vi "ActiView806-Lores.vi"() -> ()   [LabVIEW 2020] (continued)
                      tunnel: w4514 -> [w4583 w4585 w4587 w4589 w4591 w4593 w4595 w4597 w4599 w4601 w4603 w4605 w4607 w4609 w4611 w4613 w4615 w4617 w4619 w4621 w4623 w4625 w4627 w4629 w4631 w4633 w4635 w4637 w4639 w4641 w4643 w4645 w4647 w4649 w4651 w4653 w4655 w4657 w4659 w4661 w4663 w4665 w4667 w4669 w4671 w4673 w4675 w4677 w4679 w4681 w4683 w4685 w4687 w4689 w4691 w4693 w4695 w4697 w4699 w4701 w4703 w4705 w4707 w4709]
                      frame 1 {
                        n1833 = property on="Trace1" class="Str"("Position:Top"=w4583) -> ()  [unwired: 2 in, 2 out]
                        "Trace1" <- w4584
                      }
                      frame 2 {
                        n1834 = property on="Trace2" class="Str"("Position:Top"=w4585) -> ()  [unwired: 2 in, 2 out]
                        "Trace2" <- w4586
                      }
                      frame 3 {
                        n1835 = property on="Trace3" class="Str"("Position:Top"=w4587) -> ()  [unwired: 2 in, 2 out]
                        "Trace3" <- w4588
                      }
                      frame 4 {
                        n1836 = property on="Trace4" class="Str"("Position:Top"=w4589) -> ()  [unwired: 2 in, 2 out]
                        "Trace4" <- w4590
                      }
                      frame 5 {
                        n1837 = property on="Trace5" class="Str"("Position:Top"=w4591) -> ()  [unwired: 2 in, 2 out]
                        "Trace5" <- w4592
                      }
                      frame 6 {
                        n1838 = property on="Trace6" class="Str"("Position:Top"=w4593) -> ()  [unwired: 2 in, 2 out]
                        "Trace6" <- w4594
                      }
                      frame 7 {
                        n1839 = property on="Trace7" class="Str"("Position:Top"=w4595) -> ()  [unwired: 2 in, 2 out]
                        "Trace7" <- w4596
                      }
                      frame 8 {
                        n1840 = property on="Trace8" class="Str"("Position:Top"=w4597) -> ()  [unwired: 2 in, 2 out]
                        "Trace8" <- w4598
                      }
                      frame 9 {
                        n1841 = property on="Trace9" class="Str"("Position:Top"=w4599) -> ()  [unwired: 2 in, 2 out]
                        "Trace9" <- w4600
                      }
                      frame 10 {
                        n1842 = property on="Trace10" class="Str"("Position:Top"=w4601) -> ()  [unwired: 2 in, 2 out]
                        "Trace10" <- w4602
                      }
                      frame 11 {
                        n1843 = property on="Trace11" class="Str"("Position:Top"=w4603) -> ()  [unwired: 2 in, 2 out]
                        "Trace11" <- w4604
                      }
                      frame 12 {
                        n1844 = property on="Trace12" class="Str"("Position:Top"=w4605) -> ()  [unwired: 2 in, 2 out]
                        "Trace12" <- w4606
                      }
                      frame 13 {
                        n1845 = property on="Trace13" class="Str"("Position:Top"=w4607) -> ()  [unwired: 2 in, 2 out]
                        "Trace13" <- w4608
                      }
                      frame 14 {
                        n1846 = property on="Trace14" class="Str"("Position:Top"=w4609) -> ()  [unwired: 2 in, 2 out]
                        "Trace14" <- w4610
                      }
                      frame 15 {
                        n1847 = property on="Trace15" class="Str"("Position:Top"=w4611) -> ()  [unwired: 2 in, 2 out]
                        "Trace15" <- w4612
                      }
                      frame 16 {
                        n1848 = property on="Trace16" class="Str"("Position:Top"=w4613) -> ()  [unwired: 2 in, 2 out]
                        "Trace16" <- w4614
                      }
                      frame 17 {
                        n1849 = property on="Trace17" class="Str"("Position:Top"=w4615) -> ()  [unwired: 2 in, 2 out]
                        "Trace17" <- w4616
                      }
                      frame 18 {
                        n1850 = property on="Trace18" class="Str"("Position:Top"=w4617) -> ()  [unwired: 2 in, 2 out]
                        "Trace18" <- w4618
                      }
                      frame 19 {
                        n1851 = property on="Trace19" class="Str"("Position:Top"=w4619) -> ()  [unwired: 2 in, 2 out]
                        "Trace19" <- w4620
                      }
                      frame 20 {
                        n1852 = property on="Trace20" class="Str"("Position:Top"=w4621) -> ()  [unwired: 2 in, 2 out]
                        "Trace20" <- w4622
                      }
                      frame 21 {
                        n1853 = property on="Trace21" class="Str"("Position:Top"=w4623) -> ()  [unwired: 2 in, 2 out]
                        "Trace21" <- w4624
                      }
                      frame 22 {
                        n1854 = property on="Trace22" class="Str"("Position:Top"=w4625) -> ()  [unwired: 2 in, 2 out]
                        "Trace22" <- w4626
                      }
                      frame 23 {
                        n1855 = property on="Trace23" class="Str"("Position:Top"=w4627) -> ()  [unwired: 2 in, 2 out]
                        "Trace23" <- w4628
                      }
                      frame 24 {
                        n1856 = property on="Trace24" class="Str"("Position:Top"=w4629) -> ()  [unwired: 2 in, 2 out]
                        "Trace24" <- w4630
                      }
                      frame 25 {
                        n1857 = property on="Trace25" class="Str"("Position:Top"=w4631) -> ()  [unwired: 2 in, 2 out]
                        "Trace25" <- w4632
                      }
                      frame 26 {
                        n1858 = property on="Trace26" class="Str"("Position:Top"=w4633) -> ()  [unwired: 2 in, 2 out]
                        "Trace26" <- w4634
                      }
                      frame 27 {
                        n1859 = property on="Trace27" class="Str"("Position:Top"=w4635) -> ()  [unwired: 2 in, 2 out]
                        "Trace27" <- w4636
                      }
                      frame 28 {
                        n1860 = property on="Trace28" class="Str"("Position:Top"=w4637) -> ()  [unwired: 2 in, 2 out]
                        "Trace28" <- w4638
                      }
                      frame 29 {
                        n1861 = property on="Trace29" class="Str"("Position:Top"=w4639) -> ()  [unwired: 2 in, 2 out]
                        "Trace29" <- w4640
                      }
                      frame 30 {
                        n1862 = property on="Trace30" class="Str"("Position:Top"=w4641) -> ()  [unwired: 2 in, 2 out]
                        "Trace30" <- w4642
                      }
                      frame 31 {
                        n1863 = property on="Trace31" class="Str"("Position:Top"=w4643) -> ()  [unwired: 2 in, 2 out]
                        "Trace31" <- w4644
                      }
                      frame 32 {
                        n1864 = property on="Trace32" class="Str"("Position:Top"=w4645) -> ()  [unwired: 2 in, 2 out]
                        "Trace32" <- w4646
                      }
                      frame 33 {
                        n1865 = property on="Trace33" class="Str"("Position:Top"=w4647) -> ()  [unwired: 2 in, 2 out]
                        "Trace33" <- w4648
                      }
                      frame 34 {
                        n1866 = property on="Trace34" class="Str"("Position:Top"=w4649) -> ()  [unwired: 2 in, 2 out]
                        "Trace34" <- w4650
                      }
                      frame 35 {
                        n1867 = property on="Trace35" class="Str"("Position:Top"=w4651) -> ()  [unwired: 2 in, 2 out]
                        "Trace35" <- w4652
                      }
                      frame 36 {
                        n1868 = property on="Trace36" class="Str"("Position:Top"=w4653) -> ()  [unwired: 2 in, 2 out]
                        "Trace36" <- w4654
                      }
                      frame 37 {
                        n1869 = property on="Trace37" class="Str"("Position:Top"=w4655) -> ()  [unwired: 2 in, 2 out]
                        "Trace37" <- w4656
                      }
                      frame 38 {
                        n1870 = property on="Trace38" class="Str"("Position:Top"=w4657) -> ()  [unwired: 2 in, 2 out]
                        "Trace38" <- w4658
                      }
                      frame 39 {
                        n1871 = property on="Trace39" class="Str"("Position:Top"=w4659) -> ()  [unwired: 2 in, 2 out]
                        "Trace39" <- w4660
                      }
                      frame 40 {
                        n1872 = property on="Trace40" class="Str"("Position:Top"=w4661) -> ()  [unwired: 2 in, 2 out]
                        "Trace40" <- w4662
                      }
                      frame 41 {
                        n1873 = property on="Trace41" class="Str"("Position:Top"=w4663) -> ()  [unwired: 2 in, 2 out]
                        "Trace41" <- w4664
                      }
                      frame 42 {
                        n1874 = property on="Trace42" class="Str"("Position:Top"=w4665) -> ()  [unwired: 2 in, 2 out]
                        "Trace42" <- w4666
                      }
                      frame 43 {
                        n1875 = property on="Trace43" class="Str"("Position:Top"=w4667) -> ()  [unwired: 2 in, 2 out]
                        "Trace43" <- w4668
                      }
                      frame 44 {
                        n1876 = property on="Trace44" class="Str"("Position:Top"=w4669) -> ()  [unwired: 2 in, 2 out]
                        "Trace44" <- w4670
                      }
                      frame 45 {
                        n1877 = property on="Trace45" class="Str"("Position:Top"=w4671) -> ()  [unwired: 2 in, 2 out]
                        "Trace45" <- w4672
                      }
                      frame 46 {
                        n1878 = property on="Trace46" class="Str"("Position:Top"=w4673) -> ()  [unwired: 2 in, 2 out]
                        "Trace46" <- w4674
                      }
                      frame 47 {
                        n1879 = property on="Trace47" class="Str"("Position:Top"=w4675) -> ()  [unwired: 2 in, 2 out]
                        "Trace47" <- w4676
                      }
                      frame 48 {
                        n1880 = property on="Trace48" class="Str"("Position:Top"=w4677) -> ()  [unwired: 2 in, 2 out]
                        "Trace48" <- w4678
                      }
                      frame 49 {
                        n1881 = property on="Trace49" class="Str"("Position:Top"=w4679) -> ()  [unwired: 2 in, 2 out]
                        "Trace49" <- w4680
                      }
                      frame 50 {
                        n1882 = property on="Trace50" class="Str"("Position:Top"=w4681) -> ()  [unwired: 2 in, 2 out]
                        "Trace50" <- w4682
                      }
                      frame 51 {
                        n1883 = property on="Trace51" class="Str"("Position:Top"=w4683) -> ()  [unwired: 2 in, 2 out]
                        "Trace51" <- w4684
                      }
                      frame 52 {
                        n1884 = property on="Trace52" class="Str"("Position:Top"=w4685) -> ()  [unwired: 2 in, 2 out]
                        "Trace52" <- w4686
                      }
                      frame 53 {
                        n1885 = property on="Trace53" class="Str"("Position:Top"=w4687) -> ()  [unwired: 2 in, 2 out]
                        "Trace53" <- w4688
                      }
                      frame 54 {
                        n1886 = property on="Trace54" class="Str"("Position:Top"=w4689) -> ()  [unwired: 2 in, 2 out]
                        "Trace54" <- w4690
                      }
                      frame 55 {
                        n1887 = property on="Trace55" class="Str"("Position:Top"=w4691) -> ()  [unwired: 2 in, 2 out]
                        "Trace55" <- w4692
                      }
                      frame 56 {
                        n1888 = property on="Trace56" class="Str"("Position:Top"=w4693) -> ()  [unwired: 2 in, 2 out]
                        "Trace56" <- w4694
                      }
                      frame 57 {
                        n1889 = property on="Trace57" class="Str"("Position:Top"=w4695) -> ()  [unwired: 2 in, 2 out]
                        "Trace57" <- w4696
                      }
                      frame 58 {
                        n1890 = property on="Trace58" class="Str"("Position:Top"=w4697) -> ()  [unwired: 2 in, 2 out]
                        "Trace58" <- w4698
                      }
                      frame 59 {
                        n1891 = property on="Trace59" class="Str"("Position:Top"=w4699) -> ()  [unwired: 2 in, 2 out]
                        "Trace59" <- w4700
                      }
                      frame 60 {
                        n1892 = property on="Trace60" class="Str"("Position:Top"=w4701) -> ()  [unwired: 2 in, 2 out]
                        "Trace60" <- w4702
                      }
                      frame 61 {
                        n1893 = property on="Trace61" class="Str"("Position:Top"=w4703) -> ()  [unwired: 2 in, 2 out]
                        "Trace61" <- w4704
                      }
                      frame 62 {
                        n1894 = property on="Trace62" class="Str"("Position:Top"=w4705) -> ()  [unwired: 2 in, 2 out]
                        "Trace62" <- w4706
                      }
                      frame 63 {
                        n1895 = property on="Trace63" class="Str"("Position:Top"=w4707) -> ()  [unwired: 2 in, 2 out]
                        "Trace63" <- w4708
                      }
                      frame 64, Default {
                        n1896 = property on="Trace64" class="Str"("Position:Top"=w4709) -> ()  [unwired: 2 in, 2 out]
                        "Trace64" <- w4710
                      }
                    }
                  }
                }
              }
              n1897 = Unbundle By Name(w3609) -> ("LoBatChange"=w3703:bool, "JazzLoBatChange"=w3362:bool)
              n1898 = Array Size(array=w3660) -> (size(s)=w3725:i32)
              n1899 = Array Size(array=w3414) -> (size(s)=w3590:i32)
              n1900 = Array Size(array=w3716) -> (size(s)=w3724:i32)
              n1901 = Array Size(array=w3695) -> (size(s)=w3697:i32)
              n1902 = property on="RefFree" class="LstBox (strict)"("Disabled"=w3726) -> ()  [unwired: 2 in, 2 out]
              n1903 = Unbundle By Name(w3394) -> ("Sweeping"=→"Sweeping":bool, "RejAbs"=→"RejAbs":bool, "RejDif"=→"RejDif":bool)
              n1904 = Not Equal?(x=w3725, y=w3724) -> (x != y?=w3721:bool)
              n1905 = Not Equal?(x=w3590, y=w3697) -> (x != y?=w3690:bool)
              n1906 = Not Equal?(x=w3660, y=w3716) -> (x != y?=w3723:bool[])
              n1907 = Not Equal?(x=w3414, y=w3695) -> (x != y?=w3696:bool[])
              n1908 = Or Array Elements(Boolean array=w3723) -> (logical OR=w3722:bool)
              n1909 = Or Array Elements(Boolean array=w3696) -> (logical OR=w3691:bool)
              n1910 = Compound Arithmetic op=OR(w3691, w3690, w3431) -> (w3689:bool)
              n1911 = case shown="True" w3689 {
                tunnel: w3448 -> [_ w4341]
                tunnel: w3414 -> [_ w4352]
                tunnel: w3590 -> [_ w4344]
                tunnel: w3381 -> [_ w4349]
                frame False {
                }
                frame True {
                  w4343 = 8  # Nr of Bip Labels
                  w4351 = -305.0  # Upper Y-value
                  w4354 = 519.0  # Lower Y-value
                  n1912 = Not Equal To 0?(x=w4344) -> (x != 0?=w4346:bool)
                  n1913 = Increment(x=w4344) -> (x+1=w4345:i32)
                  n1914 = Subtract(x=w4354, y=w4351) -> (x-y=w4353:dbl)
                  n1915 = Select(t=w4345, s=w4346, f=2) -> (s? t:f=w4342:i32)
                  n1916 = To Double Precision Float(number=w4342) -> (double precision float=w4348:dbl)
                  n1917 = Divide(x=w4353, y=w4348) -> (x/y=w4350:dbl)
                  n1918 = for {
                    N: w4343 -> [_]
                    tunnel: w4341 -> [w4359]
                    tunnel: w4352 -> [w4365]
                    tunnel: w4351 -> [w4362]
                    tunnel: w4350 -> [w4361]
                    tunnel: w4349 -> [w4363]
                    tunnel: w4344 -> [w4366]
                    i -> [w4364]
                    n1919 = Greater?(x=w4366, y=w4364) -> (0:w4356:bool)
                    n1920 = Increment(x=w4364) -> (x+1=w4360:i32)
                    n1921 = case shown="True" w4356 {
                      tunnel: w4362 -> [_ w4391]
                      tunnel: w4361 -> [_ w4390]
                      tunnel: w4359 -> [_ w4388]
                      tunnel: w4360 -> [_ w4383]
                      tunnel: ["" w4382] -> w4358
                      tunnel: [0 w4381] -> w4357
                      tunnel: w4363 -> [_ w4374]
                      tunnel: w4365 -> [_ w4380]
                      tunnel: w4364 -> [_ w4379]
                      frame False {
                      }
                      frame True {
                        w4384 = "\r"
                        w4387 = 4 ("length (rest)")
                        n1922 = Index Array(array=w4380, index=w4379) -> (element=w4371:i32)
                        n1923 = Increment(x=w4371) -> (x+1=w4370:i32)
                        n1924 = Less?(x=w4370, y=w4374) -> (x < y?=w4376:bool)
                        n1925 = Subtract(x=w4374, y=8) -> (x-y=w4372:i32)
                        n1926 = Select(t=w4370, s=w4376, f=w4372) -> (s? t:f=w4375:i32)
                        n1927 = To Double Precision Float(number=w4383) -> (double precision float=w4389:dbl)
                        n1928 = Index Array(array=w4388, index=w4371) -> (element=w4386:string)
                        n1929 = Index Array(array=w4388, index=w4375) -> (element=w4385:string)
                        n1930 = Multiply(x=w4390, y=w4389) -> (x*y=w4392:dbl)
                        n1931 = Add(x=w4391, y=w4392) -> (x+y=w4393:dbl)
                        n1932 = String Subset(string=w4386, length (rest)=w4387) -> (substring=w4378:string)  [unwired: 1 out]
                        n1933 = String Subset(string=w4385, length (rest)=w4387) -> (substring=w4377:string)  [unwired: 1 out]
                        n1934 = To Long Integer(number=w4393) -> (32bit integer=w4381:i32)
                        n1935 = Concatenate Strings(w4378, w4384, " versus " ("Substring"), w4384, w4377) -> (w4382:string)
                      }
                    }
                    n1936 = case shown="8, Default" w4360 {
                      tunnel: w4358 -> [w4394 w4396 w4398 w4400 w4402 w4404 w4406 w4408]
                      tunnel: w4357 -> [w4395 w4397 w4399 w4401 w4403 w4405 w4407 w4409]
                      frame 1 {
                        n1937 = property on="Bip1" class="Str"("Position:Top"=w4395) -> ()  [unwired: 2 in, 2 out]
                        "Bip1" <- w4394
                      }
                      frame 2 {
                        n1938 = property on="Bip2" class="Str"("Position:Top"=w4397) -> ()  [unwired: 2 in, 2 out]
                        "Bip2" <- w4396
                      }
                      frame 3 {
                        n1939 = property on="Bip3" class="Str"("Position:Top"=w4399) -> ()  [unwired: 2 in, 2 out]
                        "Bip3" <- w4398
                      }
                      frame 4 {
                        n1940 = property on="Bip4" class="Str"("Position:Top"=w4401) -> ()  [unwired: 2 in, 2 out]
                        "Bip4" <- w4400
                      }
                      frame 5 {
                        n1941 = property on="Bip5" class="Str"("Position:Top"=w4403) -> ()  [unwired: 2 in, 2 out]
                        "Bip5" <- w4402
                      }
                      frame 6 {
                        n1942 = property on="Bip6" class="Str"("Position:Top"=w4405) -> ()  [unwired: 2 in, 2 out]
                        "Bip6" <- w4404
                      }
                      frame 7 {
                        n1943 = property on="Bip7" class="Str"("Position:Top"=w4407) -> ()  [unwired: 2 in, 2 out]
                        "Bip7" <- w4406
                      }
                      frame 8, Default {
                        n1944 = property on="Bip8" class="Str"("Position:Top"=w4409) -> ()  [unwired: 2 in, 2 out]
                        "Bip8" <- w4408
                      }
                    }
                  }
                  n1945 = To Double Precision Float(number=w4342) -> (double precision float=w4355:dbl)
                  n1946 = property on="Bip Chart" class="WFChart (strict)"("YScale.Maximum"=w4355) -> ()  [unwired: 2 in, 2 out]
                }
              }
              n1947 = Compound Arithmetic op=OR(w3722, w3721, w3692) -> (w3638:bool)
              n1948 = Not(x=w3373) -> (.not. x?=w3685:bool)
              n1949 = Array Size(array=w3660) -> (size(s)=w3734:i32)
              n1950 = global read "JazzLoBatWarning.glb" "JazzLoBatWarning"() -> (w3363:bool)
              n1951 = And(x=w3685, y=w3507) -> (x .and. y?=w3687:bool)
              "Low Battery" <- w3687
              n1952 = Equal?(x=T2."Monopolar Display" ("Charts/Graphs"), y="Charts/Graphs") -> (x = y?=w3686:bool)
              n1953 = global read "LoBatWarning.glb" "LoBatWarning"() -> (w3705:bool)
              n1954 = Equal To 0?(x=w3734) -> (x = 0?=w3581:bool)
              n1955 = Compound Arithmetic op=AND(w3686, w3581, w3685) -> (w3578:bool)
              "NoRef Blinker" <- w3578
              n1956 = call "Blinker.vi"("Ratio (>0)"=u32 5, "Period (ms)"=u32 2000, "On/Off In"=w3578) -> ("Blinker Out"=w3579:bool)
              n1957 = Not(x=w3362) -> (.not. x?=w3365:bool)
              n1958 = Not(x=w3703) -> (.not. x?=w3702:bool)
              n1959 = case shown="1, Default" w3347 {
                tunnel: w3351 -> [_ w3751]
                tunnel: [w3746 w3747] -> w3350
                tunnel: w3341 -> [w3746 w3748]
                frame 0 {
                }
                frame 1, Default {
                  # "Do not overwrite output trigger 16\n(used to switch receiver to Jazz)"
                  n1960 = Index Array(array=w3751, index (row) #1=8 ("index (row)")) -> (element #1=w3753:bool[], element #2=w3752:bool[])  [unwired: 3 in]
                  n1961 = Or Array Elements(Boolean array=w3752) -> (logical OR=w3749:bool)
                  n1962 = Or Array Elements(Boolean array=w3753) -> (logical OR=w3750:bool)
                  n1963 = Replace Array Subset(array=w3748, new element #1=w3750, new element #2=w3749) -> (w3747:bool[])  [unwired: 2 in]
                }
              }
              n1964 = property on="NoRef Blinker" class="Bool"("Visible"=w3579) -> ()  [unwired: 2 in, 2 out]
              n1965 = And(x=w3358, y=w3365) -> (x .and. y?=w3366:bool)
              n1966 = And(x=w3687, y=w3702) -> (x .and. y?=w3706:bool)
              n1967 = Or(x=w3366, y=w3363) -> (x .or. y?=w3364:bool)
              n1968 = global write "JazzLoBatWarning.glb" "JazzLoBatWarning"(w3364) -> ()
              n1969 = Or(x=w3706, y=w3705) -> (x .or. y?=w3704:bool)
              n1970 = global write "LoBatWarning.glb" "LoBatWarning"(w3704) -> ()
              n1971 = Select(t=i8 1, s=w3669, f=w3688) -> (s? t:f=w3740:i8)
              n1972 = Bundle(w3687, w3358) -> (w3707:cluster{bool, bool})  [unwired: 1 out]
              n1973 = Array Size(array=w3410) -> (size(s)=w3589:i32)
              n1974 = Array Size(array=w3651) -> (size(s)=w3655:i32)
              n1975 = stacked-sequence {
                tunnel: ["Master Filter Reset" _] -> w3493
                tunnel: ["Mon Filter Reset" _] -> w3565
                tunnel: ["Bip Filter Reset" _] -> w3564
                tunnel: ["Aux DC Reset" _] -> w3563
                tunnel: ["Ana Filter Reset" _] -> w3562
                tunnel: ["Jazz Filter Reset" _] -> w3438
                frame #0 {
                }
                frame #1 {
                  w3928 = FALSE ("Reset Sensor DC on Screen")
                  n1976 = local write "Master Filter Reset"(w3928) -> ()
                  n1977 = local write "Mon Filter Reset"(w3928) -> ()
                  n1978 = local write "Jazz Filter Reset"(w3928) -> ()
                  n1979 = local write "Ana Filter Reset"(w3928) -> ()
                  n1980 = local write "Bip Filter Reset"(w3928) -> ()
                  n1981 = local write "Aux DC Reset"(w3928) -> ()
                }
              }
              n1982 = stacked-sequence {
                tunnel: [w3885 _] -> w3560
                frame #0 {
                  n1983 = Bundle("Marker F1"="Marker F1", "Marker F2"="Marker F2", "Marker F3"="Marker F3", "Marker F4"="Marker F4", "Marker F5"="Marker F5", "Marker F6"="Marker F6", "Marker F7"="Marker F7", "Marker F8"="Marker F8") -> (w3885:T42)  [unwired: 1 out]
                }
                frame #1 {
                  w3894 = FALSE ("Reset Sensor DC on Screen")
                  n1984 = local write "Marker F1"(w3894) -> ()
                  n1985 = local write "Marker F2"(w3894) -> ()
                  n1986 = local write "Marker F3"(w3894) -> ()
                  n1987 = local write "Marker F4"(w3894) -> ()
                  n1988 = local write "Marker F5"(w3894) -> ()
                  n1989 = local write "Marker F6"(w3894) -> ()
                  n1990 = local write "Marker F7"(w3894) -> ()
                  n1991 = local write "Marker F8"(w3894) -> ()
                }
              }
              n1992 = Not Equal?(x=w3589, y=w3655) -> (x != y?=w3652:bool)
              n1993 = Not Equal?(x=w3410, y=w3651) -> (x != y?=w3654:bool[])
              n1994 = case shown="False" w3488 {
                selector: w3488 -> [_ w3823]
                tunnel: [w3819 FALSE ("Start Saving")] -> w3464
                frame False {
                  n1995 = local read "Start Saving"() -> (w3821:bool)
                  n1996 = call "AVTCP-Save FGV.vi"() -> ("Value out"=w3820:bool)  [unwired: 7 in]
                  n1997 = Or(x=w3821, y=w3820) -> (x .or. y?=w3819:bool)
                  n1998 = local write "Start Saving"(w3819) -> ()
                }
                frame True {
                  n1999 = local write "Start Saving"(w3823) -> ()
                }
              }
              n2000 = Or Array Elements(Boolean array=w3654) -> (logical OR=w3653:bool)
              n2001 = Not Equal?(x="Box", y=w3494) -> (x != y?=w3490:bool)
              n2002 = Compound Arithmetic op=OR(w3653, w3652, w3431) -> (w3648:bool)
              n2003 = case shown="True" w3648 {
                tunnel: w3589 -> [_ w3971]
                tunnel: w3448 -> [_ w3969]
                tunnel: w3410 -> [_ w3973]
                frame False {
                }
                frame True {
                  w3972 = 32  # Nr of Ana  Labels
                  w3980 = -292.0  # Upper Y-value
                  w3982 = 532.0  # Lower Y-value
                  n2004 = Not Equal To 0?(x=w3971) -> (x != 0?=w3976:bool)
                  n2005 = Increment(x=w3971) -> (x+1=w3977:i32)
                  n2006 = Subtract(x=w3982, y=w3980) -> (x-y=w3981:dbl)
                  n2007 = Select(t=w3977, s=w3976, f=2) -> (s? t:f=w3970:i32)
                  n2008 = To Double Precision Float(number=w3970) -> (double precision float=w3975:dbl)
                  n2009 = Divide(x=w3981, y=w3975) -> (x/y=w3979:dbl)
                  n2010 = for {
                    N: w3972 -> [_]
                    tunnel: w3969 -> [w3990]
                    tunnel: w3973 -> [w3987]
                    tunnel: w3980 -> [w3992]
                    tunnel: w3979 -> [w3991]
                    tunnel: w3971 -> [w3988]
                    i -> [w3983]
                    n2011 = Greater?(x=w3988, y=w3983) -> (0:w3989:bool)
                    n2012 = Increment(x=w3983) -> (x+1=w3986:i32)
                    n2013 = case shown="True" w3989 {
                      tunnel: w3992 -> [_ w4070]
                      tunnel: w3991 -> [_ w4069]
                      tunnel: w3990 -> [_ w4061]
                      tunnel: w3986 -> [_ w4065]
                      tunnel: ["" w4059] -> w3985
                      tunnel: [0 w4064] -> w3984
                      tunnel: w3987 -> [_ w4063]
                      tunnel: w3983 -> [_ w4062]
                      frame False {
                      }
                      frame True {
                        n2014 = Index Array(array=w4063, index=w4062) -> (element=w4060:i32)
                        n2015 = To Double Precision Float(number=w4065) -> (double precision float=w4068:dbl)
                        n2016 = Multiply(x=w4069, y=w4068) -> (x*y=w4071:dbl)
                        n2017 = Index Array(array=w4061, index=w4060) -> (element=w4066:string)
                        n2018 = Add(x=w4070, y=w4071) -> (x+y=w4072:dbl)
                        n2019 = String Subset(string=w4066, length (rest)=8 ("length (rest)")) -> (substring=w4059:string)  [unwired: 1 out]
                        n2020 = To Long Integer(number=w4072) -> (32bit integer=w4064:i32)
                      }
                    }
                    n2021 = case shown="32, Default" w3986 {
                      tunnel: w3985 -> [w3994 w3996 w3998 w4000 w4002 w4004 w4006 w4008 w4010 w4012 w4014 w4016 w4018 w4020 w4022 w4024 w4026 w4028 w4030 w4032 w4034 w4036 w4038 w4040 w4042 w4044 w4046 w4048 w4050 w4052 w4054 w4056]
                      tunnel: w3984 -> [w3993 w3995 w3997 w3999 w4001 w4003 w4005 w4007 w4009 w4011 w4013 w4015 w4017 w4019 w4021 w4023 w4025 w4027 w4029 w4031 w4033 w4035 w4037 w4039 w4041 w4043 w4045 w4047 w4049 w4051 w4053 w4055]
                      frame 1 {
                        n2022 = property on="Ana1" class="Str"("Position:Top"=w3993) -> ()  [unwired: 2 in, 2 out]
                        "Ana1" <- w3994
                      }
                      frame 2 {
                        n2023 = property on="Ana2" class="Str"("Position:Top"=w3995) -> ()  [unwired: 2 in, 2 out]
                        "Ana2" <- w3996
                      }
                      frame 3 {
                        n2024 = property on="Ana3" class="Str"("Position:Top"=w3997) -> ()  [unwired: 2 in, 2 out]
                        "Ana3" <- w3998
                      }
                      frame 4 {
                        n2025 = property on="Ana4" class="Str"("Position:Top"=w3999) -> ()  [unwired: 2 in, 2 out]
                        "Ana4" <- w4000
                      }
                      frame 5 {
                        n2026 = property on="Ana5" class="Str"("Position:Top"=w4001) -> ()  [unwired: 2 in, 2 out]
                        "Ana5" <- w4002
                      }
                      frame 6 {
                        n2027 = property on="Ana6" class="Str"("Position:Top"=w4003) -> ()  [unwired: 2 in, 2 out]
                        "Ana6" <- w4004
                      }
                      frame 7 {
                        n2028 = property on="Ana7" class="Str"("Position:Top"=w4005) -> ()  [unwired: 2 in, 2 out]
                        "Ana7" <- w4006
                      }
                      frame 8 {
                        n2029 = property on="Ana8" class="Str"("Position:Top"=w4007) -> ()  [unwired: 2 in, 2 out]
                        "Ana8" <- w4008
                      }
                      frame 9 {
                        n2030 = property on="Ana9" class="Str"("Position:Top"=w4009) -> ()  [unwired: 2 in, 2 out]
                        "Ana9" <- w4010
                      }
                      frame 10 {
                        n2031 = property on="Ana10" class="Str"("Position:Top"=w4011) -> ()  [unwired: 2 in, 2 out]
                        "Ana10" <- w4012
                      }
                      frame 11 {
                        n2032 = property on="Ana11" class="Str"("Position:Top"=w4013) -> ()  [unwired: 2 in, 2 out]
                        "Ana11" <- w4014
                      }
                      frame 12 {
                        n2033 = property on="Ana12" class="Str"("Position:Top"=w4015) -> ()  [unwired: 2 in, 2 out]
                        "Ana12" <- w4016
                      }
                      frame 13 {
                        n2034 = property on="Ana13" class="Str"("Position:Top"=w4017) -> ()  [unwired: 2 in, 2 out]
                        "Ana13" <- w4018
                      }
                      frame 14 {
                        n2035 = property on="Ana14" class="Str"("Position:Top"=w4019) -> ()  [unwired: 2 in, 2 out]
                        "Ana14" <- w4020
                      }
                      frame 15 {
                        n2036 = property on="Ana15" class="Str"("Position:Top"=w4021) -> ()  [unwired: 2 in, 2 out]
                        "Ana15" <- w4022
                      }
                      frame 16 {
                        n2037 = property on="Ana16" class="Str"("Position:Top"=w4023) -> ()  [unwired: 2 in, 2 out]
                        "Ana16" <- w4024
                      }
                      frame 17 {
                        n2038 = property on="Ana17" class="Str"("Position:Top"=w4025) -> ()  [unwired: 2 in, 2 out]
                        "Ana17" <- w4026
                      }
                      frame 18 {
                        n2039 = property on="Ana18" class="Str"("Position:Top"=w4027) -> ()  [unwired: 2 in, 2 out]
                        "Ana18" <- w4028
                      }
                      frame 19 {
                        n2040 = property on="Ana19" class="Str"("Position:Top"=w4029) -> ()  [unwired: 2 in, 2 out]
                        "Ana19" <- w4030
                      }
                      frame 20 {
                        n2041 = property on="Ana20" class="Str"("Position:Top"=w4031) -> ()  [unwired: 2 in, 2 out]
                        "Ana20" <- w4032
                      }
                      frame 21 {
                        n2042 = property on="Ana21" class="Str"("Position:Top"=w4033) -> ()  [unwired: 2 in, 2 out]
                        "Ana21" <- w4034
                      }
                      frame 22 {
                        n2043 = property on="Ana22" class="Str"("Position:Top"=w4035) -> ()  [unwired: 2 in, 2 out]
                        "Ana22" <- w4036
                      }
                      frame 23 {
                        n2044 = property on="Ana23" class="Str"("Position:Top"=w4037) -> ()  [unwired: 2 in, 2 out]
                        "Ana23" <- w4038
                      }
                      frame 24 {
                        n2045 = property on="Ana24" class="Str"("Position:Top"=w4039) -> ()  [unwired: 2 in, 2 out]
                        "Ana24" <- w4040
                      }
                      frame 25 {
                        n2046 = property on="Ana25" class="Str"("Position:Top"=w4041) -> ()  [unwired: 2 in, 2 out]
                        "Ana25" <- w4042
                      }
                      frame 26 {
                        n2047 = property on="Ana26" class="Str"("Position:Top"=w4043) -> ()  [unwired: 2 in, 2 out]
                        "Ana26" <- w4044
                      }
                      frame 27 {
                        n2048 = property on="Ana27" class="Str"("Position:Top"=w4045) -> ()  [unwired: 2 in, 2 out]
                        "Ana27" <- w4046
                      }
                      frame 28 {
                        n2049 = property on="Ana28" class="Str"("Position:Top"=w4047) -> ()  [unwired: 2 in, 2 out]
                        "Ana28" <- w4048
                      }
                      frame 29 {
                        n2050 = property on="Ana29" class="Str"("Position:Top"=w4049) -> ()  [unwired: 2 in, 2 out]
                        "Ana29" <- w4050
                      }
                      frame 30 {
                        n2051 = property on="Ana30" class="Str"("Position:Top"=w4051) -> ()  [unwired: 2 in, 2 out]
                        "Ana30" <- w4052
                      }
                      frame 31 {
                        n2052 = property on="Ana31" class="Str"("Position:Top"=w4053) -> ()  [unwired: 2 in, 2 out]
                        "Ana31" <- w4054
                      }
                      frame 32, Default {
                        n2053 = property on="Ana32" class="Str"("Position:Top"=w4055) -> ()  [unwired: 2 in, 2 out]
                        "Ana32" <- w4056
                      }
                    }
                  }
                  n2054 = To Double Precision Float(number=w3970) -> (double precision float=w3974:dbl)
                  n2055 = property on="Ana Chart" class="WFChart (strict)"("YScale.Maximum"=w3974) -> ()  [unwired: 2 in, 2 out]
                }
              }
              n2056 = Not(x=w3431) -> (.not. x?=w3435:bool)
              n2057 = And(x=w3490, y=w3435) -> (x .and. y?=w3489:bool)
              n2058 = Or(x=w3489, y=w3493) -> (x .or. y?=w3492:bool)
              n2059 = And(x=w3638, y=w3435) -> (x .and. y?=w3577:bool)
              n2060 = And(x=w3689, y=w3435) -> (x .and. y?=w3573:bool)
              n2061 = And(x=w3591, y=w3435) -> (x .and. y?=w3574:bool)
              n2062 = And(x=w3435, y=w3433) -> (x .and. y?=w3436:bool)
              n2063 = And(x=w3435, y=w3648) -> (x .and. y?=w3575:bool)
              n2064 = case shown="\"Jazz Eyetracker\"" "Charts/Graphs" {
                tunnel: w3577 -> [w3900 _ _ _ _ _]
                tunnel: w3565 -> [w3899 _ _ _ _ _]
                tunnel: [w3898 w3901 w3906 w3911 w3916 w3921] -> w3576
                tunnel: w3575 -> [_ _ _ _ w3920 _]
                tunnel: w3562 -> [_ _ _ _ w3919 _]
                tunnel: w3574 -> [_ _ w3910 _ _ _]
                tunnel: w3563 -> [_ _ w3909 _ _ _]
                tunnel: w3573 -> [_ w3905 _ _ _ _]
                tunnel: w3564 -> [_ w3904 _ _ _ _]
                tunnel: [w3896 w3903 w3906 w3911 w3916 w3921] -> w3572
                tunnel: [w3896 w3901 w3906 w3911 w3918 w3921] -> w3571
                tunnel: [w3896 w3901 w3908 w3911 w3916 w3921] -> w3570
                tunnel: w3492 -> [w3897 w3902 w3907 w3915 w3917 _]
                tunnel: [w3896 w3901 w3906 w3912 w3916 w3921] -> w3439
                tunnel: w3438 -> [_ _ _ w3913 _ _]
                tunnel: w3436 -> [_ _ _ w3914 _ _]
                frame "Monopolar Display" {
                  w3896 = FALSE
                  n2065 = Compound Arithmetic op=OR(w3897, w3899, w3900) -> (w3898:bool)
                }
                frame "Bipolar Leads" {
                  w3901 = FALSE
                  n2066 = Compound Arithmetic op=OR(w3902, w3904, w3905) -> (w3903:bool)
                }
                frame "Auxiliary Sensors" {
                  w3906 = FALSE
                  n2067 = Compound Arithmetic op=OR(w3907, w3909, w3910) -> (w3908:bool)
                }
                frame "Jazz Eyetracker" {
                  w3911 = FALSE
                  n2068 = Compound Arithmetic op=OR(w3915, w3913, w3914) -> (w3912:bool)
                }
                frame "Analog Input Box" {
                  w3916 = FALSE
                  n2069 = Compound Arithmetic op=OR(w3917, w3919, w3920) -> (w3918:bool)
                }
                frame "About ActiView", Default {
                  w3921 = FALSE
                }
              }
              n2070 = call "Act_Error_Jazz.vi"("Error Code In"=w3372, "error in (no error)"=w3536) -> ("error out"=w3662:errorcluster)  [unwired: 2 out]
              n2071 = Or(x=w3466, y=w3464) -> (x .or. y?=w3465:bool)
            }
            frame 2 {
              w4730 = 0.0 ("XScale.Maximum")
              w4773 = i64 0 ("Prop Screen Minimum")
              # "Save Blocksize in Bytes"
              # "Nr of Saved Bytes"
              # "Write Error"
              # "New Total Saved in Sec"
              # "Old Total Saved in Sec"
              # "Index"
              # "Save Buffer"
              # "Second Half ?"
              # "Save Blocksize in Bytes"
              # "Pause Saving"
              # "Bytes, 3 per Channel"
              # "Save"
              # "Header Lenght in Byte"
              # "Nr of Byte Saved in this Scan"
              # "New Current File in Byte"
              # "Old Current File in Byte"
              n2072 = Select(t=w4733, s=w4747, f=0) -> (s? t:f=w4746:i32)
              n2073 = Not(x=w4747) -> (.not. x?=w4750:bool)
              n2074 = Select(t=0, s=w4743, f=w4733) -> (s? t:f=w4744:i32)
              n2075 = Array Subset(array=w4749, index=w4746, length=w4744) -> (w4748:u8[])
              n2076 = Array Size(array=w4748) -> (size(s)=w4752:i32)
              n2077 = case shown="0" w4753 {
                tunnel: w4754 -> [w4805 w4811]
                tunnel: w4751 -> [w4804 w4810]
                tunnel: [w4803 w4810] -> w4741
                tunnel: [w4802 w4811] -> w4740
                frame 0 {
                  n2078 = Get Date/Time In Seconds() -> (seconds since 1Jan1904=w4798:timestamp)
                  n2079 = To Double Precision Float(number=w4798) -> (double precision float=w4800:dbl)
                  n2080 = Decrement(x=w4800) -> (x-1=w4799:dbl)
                  n2081 = Format Date/Time String(time format string (%c)="%d.%m.%y%H.%M.%S", seconds (now)=w4799) -> (date/time string=w4797:string)  [unwired: 1 out]
                  n2082 = Format Into String(format string="%-16.16s", w4797) -> (resulting string=w4806:string)  [unwired: 2 in, 1 out]
                  n2083 = call "Write File+ [String].vi"("String"=w4806, "error in (no error)"=w4804, "pos offset (bytes:0)"=i64 168, "pos mode (rel. to end:1)"=enum16{"start", "end", "current"}."start", "refnum"=w4805) -> ("error out"=w4803:errorcluster, "dup refnum"=w4802:refnum<file>)  [unwired: 2 out]
                }
                frame 1, Default {
                }
              }
              n2084 = call "Write File+ [U8].vi"("1D array"=w4748, "error in (no error)"=w4741, "refnum"=w4740) -> ("error out"=w4792:errorcluster, "dup refnum"=w4735:refnum<file>)  [unwired: 2 in, 2 out]
              n2085 = Unbundle By Name(w4792) -> ("status"=w4756:bool)
              n2086 = Select(t=0, s=w4756, f=w4752) -> (s? t:f=w4759:i32)
              n2087 = To Quad Integer(1:w4759) -> (0:w4738:i64)
              n2088 = Refnum to Path(1:w4735) -> (0:w4736:path)
              n2089 = Add(x=w4785, y=w4738) -> (x+y=w4769:i64)
              n2090 = Get Volume Info(11:w4736) -> (1:w4734:i64)  [unwired: 1 in, 5 out]
              n2091 = To Quad Integer(1:w4733) -> (0:w4732:i64)
              n2092 = Quotient & Remainder(x=w4734, y=w4732) -> (floor(x/y)=→"Free on Disk sec":i64)  [unwired: 1 out]
              n2093 = Quotient & Remainder(x=w4759, y=w4733) -> (floor(x/y)=w4758:i32)  [unwired: 1 out]
              n2094 = Add(x=w4753, y=w4758) -> (x+y=w4757:i32)
              n2095 = Scale By Power Of 2(n=i16 20, x=1.0) -> (x*2^n=w4789:dbl)
              n2096 = To Double Precision Float(number=w4769) -> (double precision float=w4787:dbl)
              n2097 = Divide(x=w4787, y=w4789) -> (x/y=→"Current File MB":dbl)
            }
            frame 3 {
              w4815 = 0.0 ("XScale.Maximum")
              w4826 = 1000  # Max Nr of Files
              w4852 = i64 0 ("Prop Screen Minimum")
              # "Start New File ?"
              # "File Error"
              # "Save Blocksize in Byte"
              # "Current File in Byte"
              # "Header Lenght in Byte"
              # "End of File"
              n2098 = Not(x=w4830) -> (.not. x?=w4827:bool)
              n2099 = Add(x=w4822, y=w4818) -> (x+y=w4821:i32)
              n2100 = To Quad Integer(1:w4821) -> (0:w4817:i64)
              n2101 = Greater Or Equal?(x=w4820, y=w4817) -> (x >= y?=w4823:bool)
              n2102 = Less?(x=w4825, y=w4826) -> (x < y?=w4824:bool)
              n2103 = Compound Arithmetic op=AND(w4823, w4824, "FileAppend", w4827) -> (w4828:bool)
              n2104 = case shown="True" w4828 {
                tunnel: w4837 -> [w4873 w4894]
                tunnel: w4838 -> [w4874 w4893]
                tunnel: [w4873 w4901] -> w4836
                tunnel: [w4869 w4921] -> w4835
                tunnel: [w4872 w4900] -> w4834
                tunnel: w4825 -> [w4871 w4903]
                tunnel: [w4871 w4932] -> w4833
                tunnel: w4832 -> [w4870 w4923]
                tunnel: w4822 -> [_ w4895]
                tunnel: w4818 -> [_ w4922]
                tunnel: [w4870 w4878] -> w4831
                frame False {
                  w4875 = FALSE
                  w4869 = TRUE  # File at Limit Error
                  n2105 = Build Array(w4875, w4875, w4875, w4869) -> (w4876:bool[])
                  n2106 = Boolean Array To Number(Boolean array=w4876) -> (number=w4877:u32)
                  n2107 = call "Act_Error_Jazz.vi"("Error Code In"=w4877, "error in (no error)"=w4874) -> ("error out"=w4872:errorcluster)  [unwired: 2 out]
                }
                frame True {
                  # "new date/time"
                  # "Old Header"
                  # "New Current File in Byte"
                  # "Old Number of Files"
                  # "Old Path"
                  # "number of data records"
                  n2108 = To Quad Integer(1:w4895) -> (0:w4878:i64)
                  n2109 = To Quad Integer(1:w4922) -> (0:w4879:i64)
                  n2110 = Subtract(x=w4923, y=w4878) -> (x-y=w4931:i64)
                  n2111 = Quotient & Remainder(x=w4931, y=w4879) -> (floor(x/y)=w4924:i64)  [unwired: 1 out]
                  n2112 = Format Into String(format string="%-8d", w4924) -> (resulting string=w4929:string)  [unwired: 2 in, 1 out]
                  n2113 = call "Read File+ [String].vi"("count"=w4895, "error in (no error)"=w4893, "pos mode (rel. to current:2)"=enum16{"start", "end", "current"}."start", "refnum"=w4894) -> ("error out"=w4891:errorcluster, "string"=w4888:string, "dup refnum"=w4890:refnum<file>)  [unwired: 1 in, 2 out]
                  n2114 = call "Write File+ [String].vi"("String"=w4929, "error in (no error)"=w4891, "pos offset (bytes:0)"=i64 236, "pos mode (rel. to end:1)"=enum16{"start", "end", "current"}."start", "refnum"=w4890) -> ("error out"=w4928:errorcluster, "dup refnum"=w4927:refnum<file>)  [unwired: 2 out]
                  n2115 = Close File(refnum=w4927, error in=w4928) -> (path=w4904:path, error out=w4880:errorcluster)
                  n2116 = Strip Path(path=w4904) -> (stripped path=w4915:path, name=w4918:string)
                  n2117 = Greater?(x=w4903, y=1) -> (0:w4913:bool)
                  n2118 = Select(t=8 ("y"), s=w4913, f=4) -> (s? t:f=w4911:i32)
                  n2119 = String Length(string=w4918) -> (length=w4920:i32)
                  n2120 = Format Into String(format string="%03d" ("Format String"), w4903) -> (resulting string=w4908:string)  [unwired: 2 in, 1 out]
                  n2121 = Subtract(x=w4920, y=w4911) -> (x-y=w4919:i32)
                  n2122 = String Subset(string=w4918, length (rest)=w4919) -> (substring=w4917:string)  [unwired: 1 out]
                  n2123 = Concatenate Strings("+", w4908, ".bdf") -> (w4905:string)
                  n2124 = Format Date/Time String(time format string (%c)="%d.%m.%y%H.%M.%S") -> (date/time string=w4897:string)  [unwired: 2 out]
                  n2125 = Format Into String(format string="%-16.16s", w4897) -> (resulting string=w4889:string)  [unwired: 2 in, 1 out]
                  n2126 = Concatenate Strings(w4917, w4905) -> (w4916:string)
                  n2127 = Build Path(base path=w4915, name or relative path=w4916) -> (appended path=w4884:path)
                  n2128 = Path To String(path=w4884) -> (string=w4896:string)
                  n2129 = local write "Filepath"(w4896) -> ()
                  n2130 = Increment(x=w4903) -> (x+1=w4932:i32)
                  n2131 = Replace Substring(2:16 ("length (len. of substring)"), 3:i64 168 ("pos offset (bytes:0)"), 4:w4889, 5:w4888) -> (1:w4885:string)  [unwired: 1 out]
                  n2132 = Open/Create/Replace File(file path (use dialog)=w4884, error in=w4880, operation (0:open)=T10."replace or create") -> (refnum out=w4881:refnum<file>, error out=w4882:errorcluster)  [unwired: 4 out]
                  n2133 = call "Write File+ [String].vi"("String"=w4885, "error in (no error)"=w4882, "pos mode (rel. to end:1)"=enum16{"start", "end", "current"}."start", "refnum"=w4881) -> ("error out"=w4900:errorcluster, "dup refnum"=w4901:refnum<file>)  [unwired: 1 in, 2 out]
                  n2134 = Unbundle By Name(w4900) -> ("status"=w4921:bool)
                }
              }
            }
            frame 4 {
              w4967 = 1000.0 ("y")
              w4950 = 0.0 ("XScale.Maximum")
              w4964 = 2  # Nr of AVG Chan
              w4975 = i64 0 ("Prop Screen Minimum")
              # "Noise Total"
              # "Average Total"
              # "Average"
              n2135 = Unbundle By Name(w4941) -> ("Sweep Lenght in Samples"=w4943:i32, "Valid Sweeps"=→"Valid Sweeps":i32, "Rejected Sweeps"=→"Rejected Sweeps":i32, "First Graph Update"=w4942:bool)
              n2136 = To Double Precision Float(number=w4943) -> (double precision float=w4958:dbl)
              n2137 = Bundle By Name(cluster=w4941, "First Graph Update"=FALSE ("Start Averaging")) -> (w4940:T11)
              n2138 = Multiply(x=w4958, y=w4967) -> (x*y=w4968:dbl)
              n2139 = Divide(x=w4968, y=w4963) -> (x/y=w4965:dbl)
              n2140 = Divide(x=w4967, y=w4963) -> (x/y=w4966:dbl)
              n2141 = for {
                tunnel: w4947 -> [w4998] mode=indexing
                tunnel: w4946 -> [w4997] mode=indexing
                tunnel: [w4996] -> w4936 mode=indexing
                tunnel: w4958 -> [w4995]
                tunnel: [w4994] -> w4935 mode=indexing
                n2142 = Add Array Elements(numeric array=w4998) -> (sum=w4999:dbl)
                n2143 = Add Array Elements(numeric array=w4997) -> (sum=w5001:dbl)
                n2144 = Divide(x=w4999, y=w4995) -> (x/y=w5000:dbl)
                n2145 = Divide(x=w5001, y=w4995) -> (x/y=w5002:dbl)
                n2146 = Subtract(x=w4998, y=w5000) -> (x-y=w4994:dbl[])
                n2147 = Subtract(x=w4997, y=w5002) -> (x-y=w4996:dbl[])
              }
              n2148 = Array Max & Min(array=w4935) -> (max value=w4938:dbl, min value=w4937:dbl)  [unwired: 2 out]
              n2149 = for {
                N: w4964 -> [_]
                tunnel: "AvgAutoscale" -> [w5018]
                tunnel: "AvgScale" -> [w5017]
                tunnel: w4965 -> [w5015]
                tunnel: w4966 -> [w5014]
                tunnel: w4942 -> [w5011]
                tunnel: w4938 -> [w5008]
                tunnel: w4937 -> [w5007]
                tunnel: w4935 -> [w5006]
                tunnel: w4936 -> [w5005]
                i -> [w5009]
                n2150 = case shown="False" w5018 {
                  tunnel: w5008 -> [_ w5042]
                  tunnel: [w5039 w5042] -> w5013
                  tunnel: w5007 -> [_ w5041]
                  tunnel: [w5040 w5041] -> w5012
                  tunnel: w5017 -> [w5039 _]
                  frame False {
                    n2151 = Negate(x=w5039) -> (-x=w5040:dbl)
                  }
                  frame True {
                  }
                }
                n2152 = Index Array(array=w5005, index (row)=w5009) -> (element=w5003:dbl[])  [unwired: 1 in]
                n2153 = Index Array(array=w5006, index (row)=w5009) -> (element=w5004:dbl[])  [unwired: 1 in]
                n2154 = Increment(x=w5009) -> (x+1=w5016:i32)
                n2155 = Build Array(w5004, w5003) -> (w5010:dbl[][])
                n2156 = case shown="2" w5016 {
                  tunnel: w5010 -> [w5021 w5031]
                  tunnel: w5014 -> [w5023 w5033]
                  tunnel: w5015 -> [w5024 w5034]
                  tunnel: w5012 -> [w5019 w5029]
                  tunnel: w5013 -> [w5020 w5030]
                  tunnel: w5011 -> [w5022 w5032]
                  frame 1, Default {
                    n2157 = case shown="True" w5022 {
                      tunnel: w5024 -> [_ w5026]
                      tunnel: w5023 -> [_ w5025]
                      frame False {
                      }
                      frame True {
                        n2158 = stacked-sequence {
                          tunnel: w5026 -> [_ w5028]
                          tunnel: w5025 -> [w5027 _]
                          frame #0 {
                            n2159 = property on="Avg1" class="WFGraph (strict)"("X Scale.Offset and Multiplier:Multiplier"=w5027) -> ()  [unwired: 2 in, 2 out]
                          }
                          frame #1 {
                            n2160 = property on="Avg1" class="WFGraph (strict)"("X Scale.Range:Maximum"=w5028) -> ()  [unwired: 2 in, 2 out]
                          }
                        }
                      }
                    }
                    n2161 = property on="Avg1" class="WFGraph (strict)"("Y Scale.Range:Maximum"=w5020, "YScale.Minimum"=w5019) -> ()  [unwired: 2 in, 2 out]
                    "Avg1" <- w5021
                  }
                  frame 2 {
                    n2162 = case shown="True" w5032 {
                      tunnel: w5034 -> [_ w5036]
                      tunnel: w5033 -> [_ w5035]
                      frame False {
                      }
                      frame True {
                        n2163 = stacked-sequence {
                          tunnel: w5036 -> [_ w5038]
                          tunnel: w5035 -> [w5037 _]
                          frame #0 {
                            n2164 = property on="Avg2" class="WFGraph (strict)"("X Scale.Offset and Multiplier:Multiplier"=w5037) -> ()  [unwired: 2 in, 2 out]
                          }
                          frame #1 {
                            n2165 = property on="Avg2" class="WFGraph (strict)"("X Scale.Range:Maximum"=w5038) -> ()  [unwired: 2 in, 2 out]
